vi "Send State Message Over LSR.vi"(8 "error in (no error)":errorcluster, 11 "LSR Instrument in":refnum<class "LSR Instrument.lvclass">) -> (0 "error out":errorcluster, 3 "LSR Instrument out":refnum<class "LSR Instrument.lvclass">)   [LabVIEW 2015, in "LSR Instrument.lvlib" / "LSR Instrument.lvclass"]
uses:
  LSR Instrument.lvclass
  <vilib>/ActorFramework/Actor/Actor.lvclass/Actor.ctl
  <vilib>/ActorFramework/Message Enqueuer/Message Enqueuer.lvclass/Message Enqueuer.ctl
  LSR Instrument.lvclass/LSR Instrument.ctl
  LSR Instrument Messages/Send RDS Message Over LSR Msg/Send RDS Message Over LSR Msg.lvclass/Send RDS Message Over LSR Msg.ctl
  <vilib>/ActorFramework/Message Enqueuer/Init from Existing Queue.vi
  <vilib>/ActorFramework/Message Enqueuer/Enqueue.vi
  <vilib>/ActorFramework/Message Priority Queue/Priority Enqueue.vi
  <vilib>/ActorFramework/Message Enqueuer/Message Enqueuer.lvclass
  LSR Instrument Messages/Send RDS Message Over LSR Msg/Send RDS Message Over LSR Msg.lvclass
  <vilib>/ActorFramework/Actor/Actor.lvclass
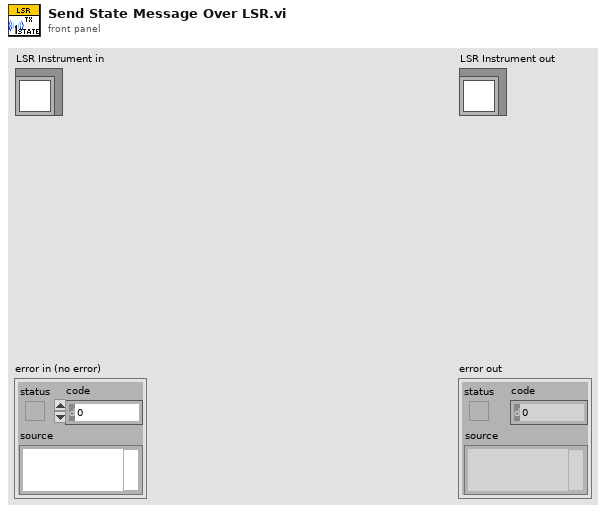
[diagram p1: front panel]
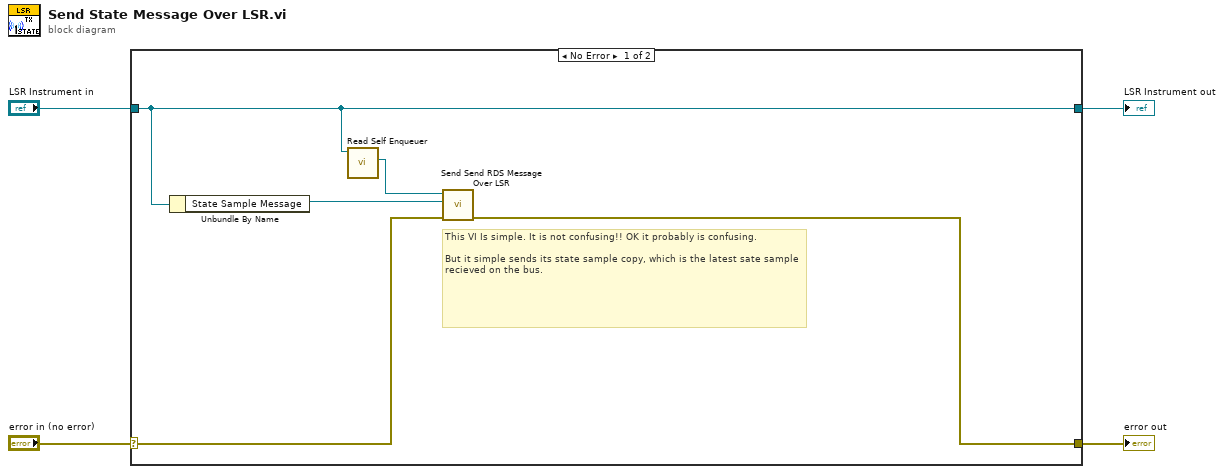
[diagram p0: block diagram]
diagram:
  n1 = case shown="No Error" "error in (no error)" {
    selector: "error in (no error)" -> [w8 w11]
    tunnel: [w7 w11] -> w3
    tunnel: [w6 w10] -> w1
    tunnel: "LSR Instrument in" -> [w6 w10]
    frame No Error {
      # "This VI Is simple. It is not confusing!! OK it probably is confusing. \n\nBut it simple sends its state sample copy, which is the latest sate sample recieved on the bus."
      n2 = Unbundle By Name(w6) -> ("State Sample Message"=w5:refnum<class "State Sample Message.lvclass">)
      n3 = call <vilib>:"Read Self Enqueuer.vi"("Actor"=w6) -> ("Self Enqueuer"=w9:refnum<class "Message Enqueuer.lvclass">)  [unwired: 10 in]
      n4 = call "Send Send RDS Message Over LSR.vi"("error in (no error)"=w8, "RDS Child Message"=w5, "Message Enqueuer"=w9) -> ("error out"=w7:errorcluster)  [unwired: 7 in, 1 out]
    }
    frame Error {
    }
  }
  "error out" <- w3
  "LSR Instrument out" <- w1
